vi "roller_globals.vi"() -> ()   [LabVIEW 2011]
panel:
  in  "sws":T1
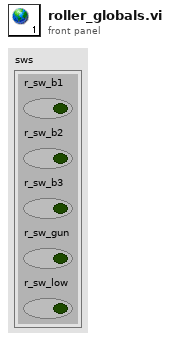
[diagram p1: front panel]
types:
  T1 = cluster{"r_sw_b1":bool, "r_sw_b2":bool, "r_sw_b3":bool, "r_sw_gun":bool, "r_sw_low":bool}
diagram:
